vi "Facade.vi"(0 "Data In":T5={"Format"=0, "Stimulus"={"Destination"="", "Rep rate (/sec)"=0.0, "Alternate Polarity"=FALSE, "Duration (ms)"=0.0, "Ramp (ms)"=16.0, "Fs (Hz)"=5.0, "Frame size (s)"=0.0}, "Sequence"={"Freq"={"Expression"="", "Step"=80}, "Level"={"Start (dB)"=20, "Stop (dB)"=80, "Step (dB)"=5}, "Order"=enum."Interleaved"}, "Response"={"Gain"=10000.0, "Averages"=512, "Window (ms)"=8.5, "Fs (Hz)"=25000.0, "Save raw"=FALSE}, "Reject"=0.0} {"Sequence"."Level"."Start (dB)" step=5; "Response"."Window (ms)" format="%.2f"}, 2 "Display State In":T3, 3 "Container State":T4) -> (6 "Data Out":T5={"Format"=0, "Stimulus"={"Destination"="", "Rep rate (/sec)"=0.0, "Alternate Polarity"=FALSE, "Duration (ms)"=0.0, "Ramp (ms)"=16.0, "Fs (Hz)"=5.0, "Frame size (s)"=0.0}, "Sequence"={"Freq"={"Expression"="", "Step"=80}, "Level"={"Start (dB)"=20, "Stop (dB)"=80, "Step (dB)"=5}, "Order"=enum."Interleaved"}, "Response"={"Gain"=10000.0, "Averages"=512, "Window (ms)"=8.5, "Fs (Hz)"=25000.0, "Save raw"=FALSE}, "Reject"=0.0} {"Sequence"."Level"."Start (dB)" step=5; "Response"."Window (ms)" format="%.2f"}, 7 "Display State Out":T3, 8 "Action":T2)   [LabVIEW 2020, in "FABR-Parameters.xctl"]
uses:
  FABR-Parameters.xctl
  Data.vi
  FABR-Stimulus.ctl
  FABR-Sequence.ctl
  FABR-Order.ctl
  FABR-Response.ctl
  <vilib>/_xctls/Container State.ctl
  State.vi
  <vilib>/_xctls/Action.ctl
  epl-vi-lib/Utility VIs/Buttons/KCheckmarkBoolean 2.ctl
  8ab337da-13bf-40eb-afaf-d46579a93e22.vi
  <vilib>/Comparison/Equal/Equal Functor/Equal Functor.lvclass
  <vilib>/_xctls/XControlSupport.lvlib
panel:
  in  "Order":enum16{"Interleaved"}(ring)
  in  "Window (ms)":sgl=8.5 format="%.2f"
  in  "Averages":i32=512
  in  "Gain":i32=10000
  in  "Step":i32
  in  "Expr":string caption="Frequency"
  in  "Alternate Polarity":T1
  in  "Rep rate (/sec)":dbl=30.0
  in  "Step (dB)":i32=5
  in  "Max (dB)":i32=80
  in  "Min (dB)":i32=20 caption="Level" step=5
  in  "Destination":u16(ring)=1 items=["Right ear", "Left ear"]
  # "Stimulus"
  # "Response"
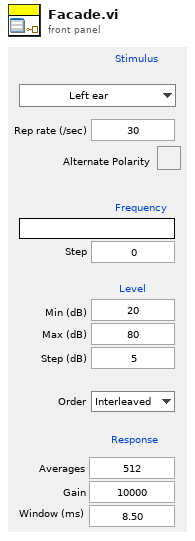
[diagram p1: front panel]
types:
  T1 = typedef "KCheckmarkBoolean 2.ctl" = bool
  T2 = typedef "XControlSupport.lvlib/Action.ctl" = cluster{"Data Changed?":bool, "State Changed?":bool, "Action Name":string}
  T3 = typedef "FABR-Parameters.xctl/State.vi" = cluster{"action":string, "destinations":string[]}
  T4 = typedef "XControlSupport.lvlib/Container State.ctl" = cluster{"Indicator?":bool, "Run Mode?":bool, " Refnum":refnum<vi>}
  T5 = typedef "FABR-Parameters.xctl/Data.vi" = cluster{"Format":i32, "Stimulus":T6, "Sequence":T7, "Response":T9, "Reject":dbl}
  T6 = typedef "FABR-Stimulus.ctl" = cluster{"Destination":string, "Rep rate (/sec)":dbl, "Alternate Polarity":bool, "Duration (ms)":dbl, "Ramp (ms)":dbl, "Fs (Hz)":dbl, "Frame size (s)":dbl}
  T7 = typedef "FABR-Sequence.ctl" = cluster{"Freq":cluster{"Expression":string, "Step":i32}, "Level":cluster{"Start (dB)":i32, "Stop (dB)":i32, "Step (dB)":i32}, "Order":T8}
  T8 = typedef "FABR-Order.ctl" = enum16{"Interleaved"}
  T9 = typedef "FABR-Response.ctl" = cluster{"Gain":dbl, "Averages":i32, "Window (ms)":sgl, "Fs (Hz)":dbl, "Save raw":bool}
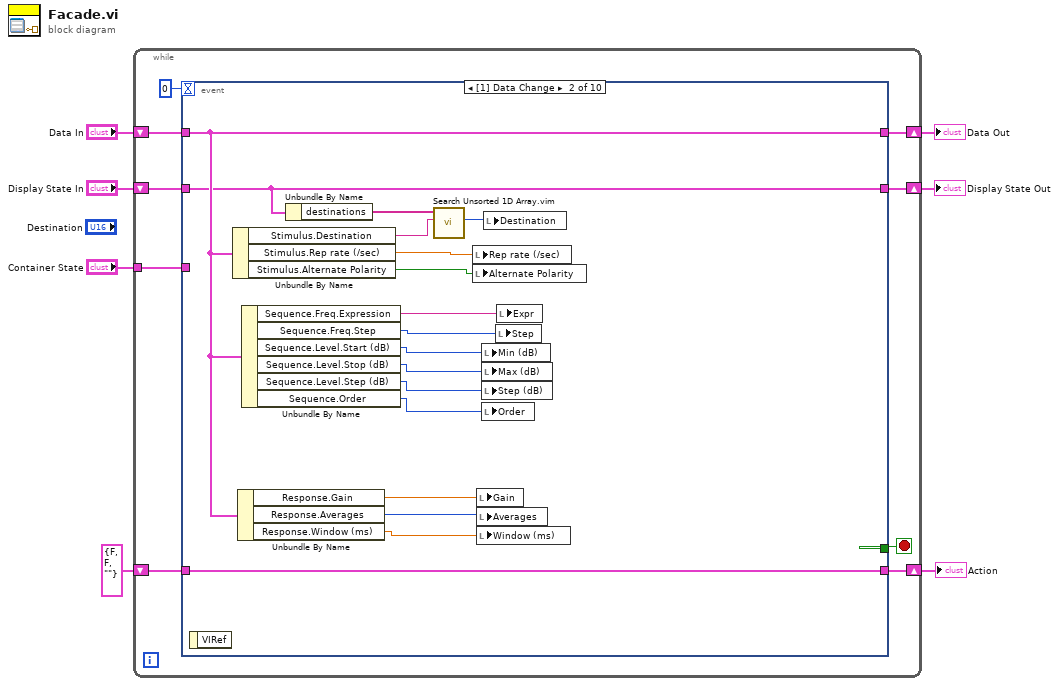
[diagram p0: block diagram]
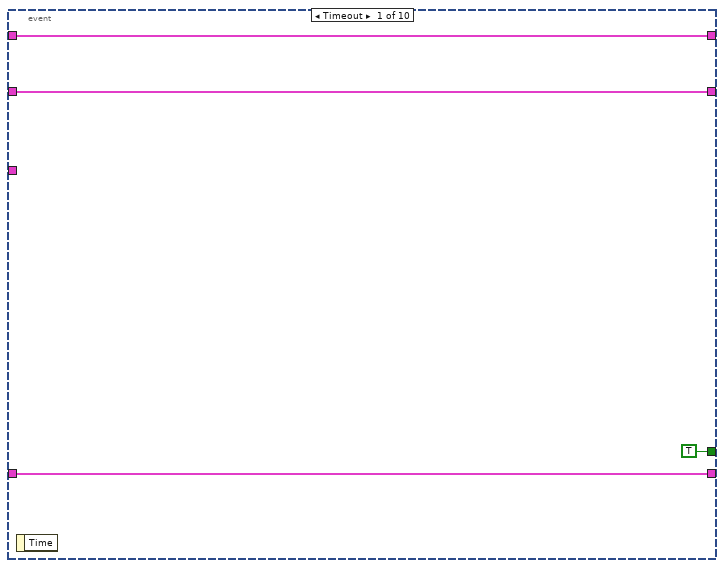
[diagram p2: hidden frame]
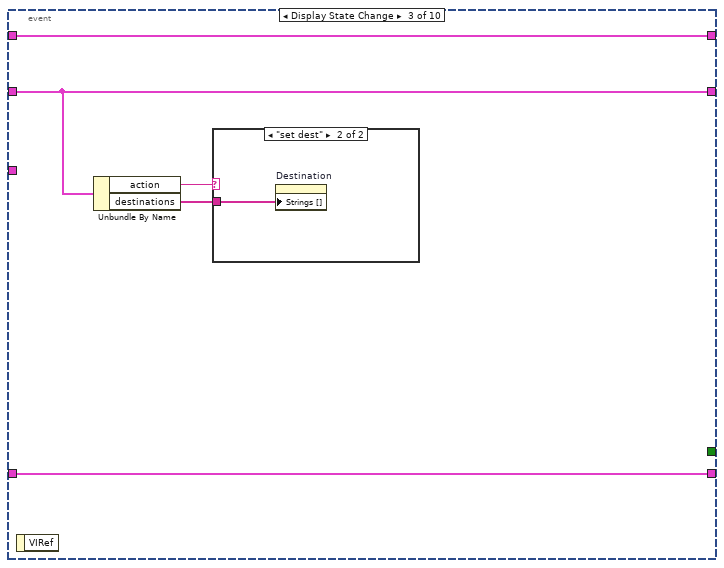
[diagram p3: hidden frame]
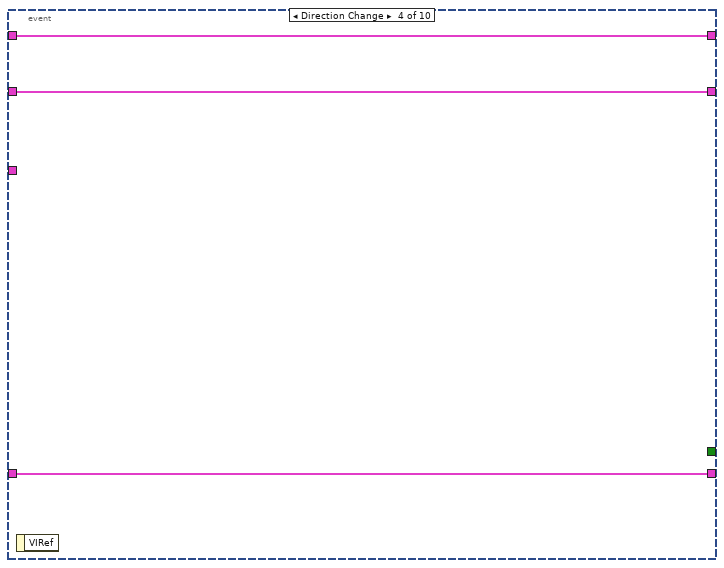
[diagram p5: hidden frame]
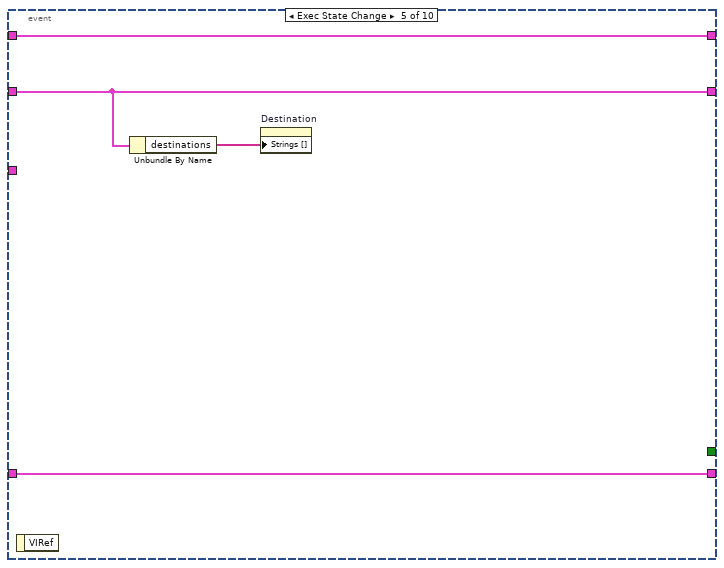
[diagram p6: hidden frame]
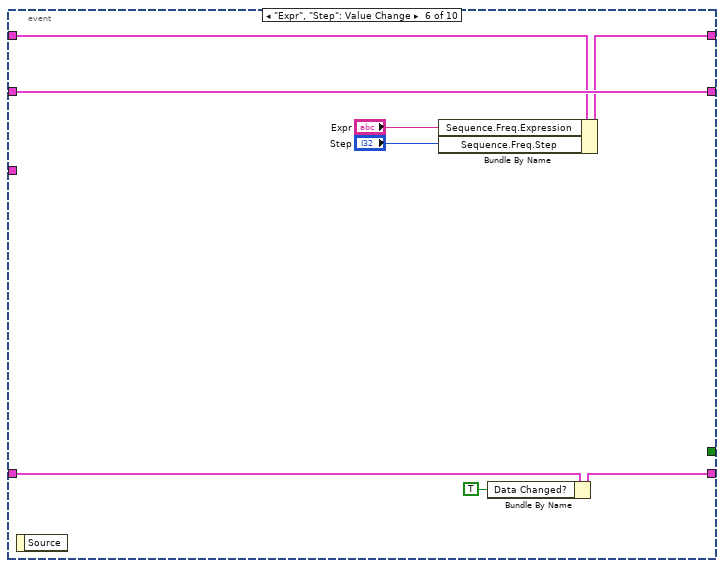
[diagram p7: hidden frame]
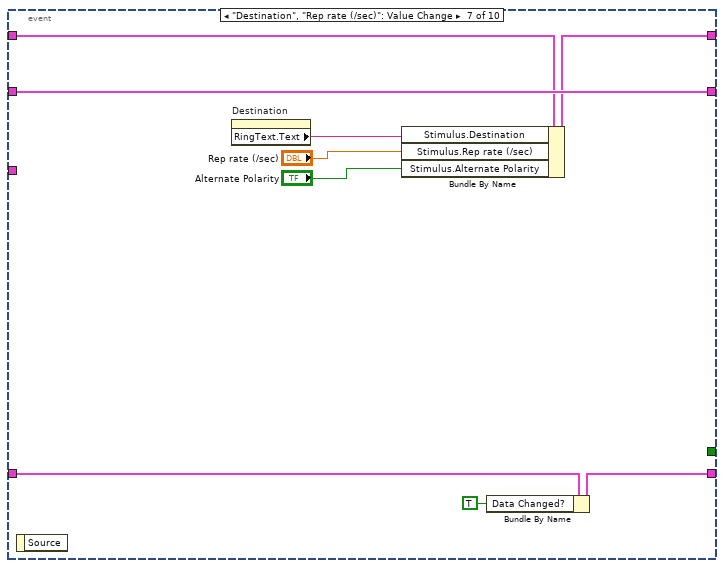
[diagram p8: hidden frame]
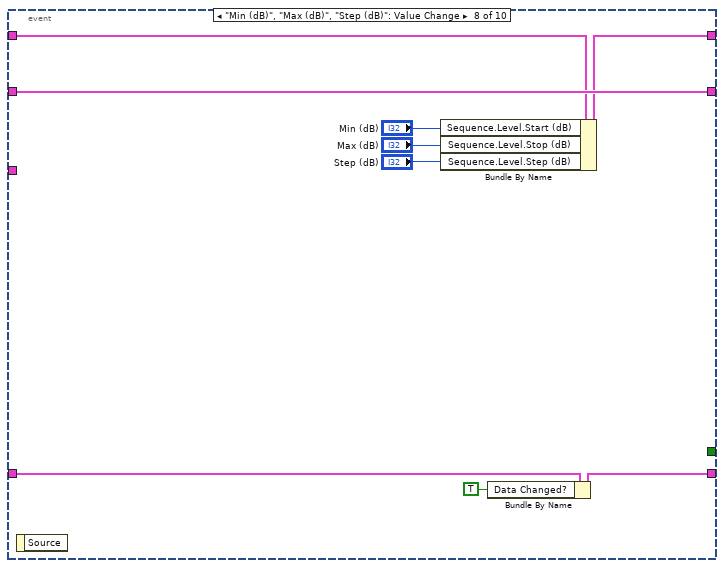
[diagram p9: hidden frame]
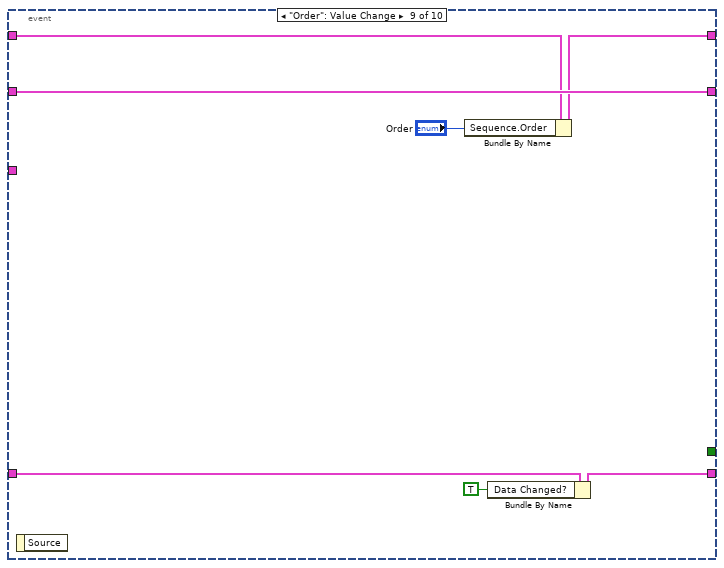
[diagram p10: hidden frame]
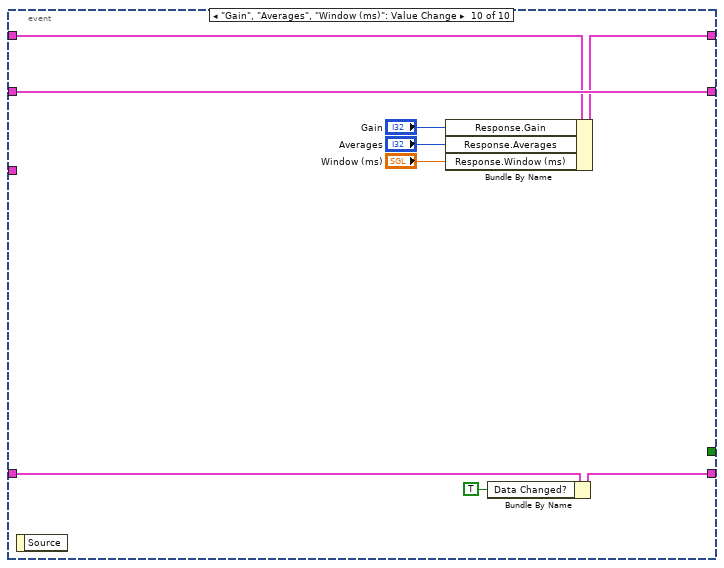
[diagram p11: hidden frame]
diagram:
  n1 = while {
    shift-right: [w15] -> w4
    shift-left: "Display State In" -> [w16]
    tunnel: "Container State" -> [w12]
    shift-right: [w10] -> w7
    shift-left: "Data In" -> [w11]
    shift-right: [w8] -> w2
    shift-left: T2 {"Data Changed?"=FALSE, "State Changed?"=FALSE, "Action Name"=""} ("Action") -> [w9]
    stop <- w14 stop-if-true
    n2 = event shown="[1] Data Change" {
      selector: _ -> [_ _ _ _ _ _ _ _ _ _]
      dyn-events: _ -> [_ _ _ _ _ _ _ _ _ _]
      timeout: 0 -> [_ _ _ _ _ _ _ _ _ _]
      tunnel: w16 -> [w18 w24 w40 w46 w48 w58 w67 w76 w83 w92]
      tunnel: [w18 w24 w40 w46 w48 w58 w67 w76 w83 w92] -> w15
      tunnel: [TRUE _ _ _ _ _ _ _ _ _] -> w14
      tunnel: w12 -> [_ _ _ _ _ _ _ _ _ _]
      tunnel: w11 -> [w17 w28 w42 w45 w50 w57 w66 w75 w82 w91]
      tunnel: [w17 w28 w42 w45 w50 w53 w62 w71 w78 w87] -> w10
      tunnel: [w19 w37 w41 w44 w49 w55 w64 w73 w80 w89] -> w8
      tunnel: w9 -> [w19 w37 w41 w44 w49 w56 w65 w74 w81 w90]
      event Timeout {
        n3 = event-data() -> ()  [unwired: 1 in, 1 out]
      }
      event Data Change {
        n4 = event-data() -> ()  [unwired: 1 in, 1 out]
        n5 = Unbundle By Name(w28) -> ("Stimulus.Destination"=w22:string, "Stimulus.Rep rate (/sec)"=w36:dbl, "Stimulus.Alternate Polarity"=w35:bool)
        n6 = Unbundle By Name(w28) -> ("Response.Gain"=w27:dbl, "Response.Averages"=w26:i32, "Response.Window (ms)"=w25:sgl)
        n7 = Unbundle By Name(w28) -> ("Sequence.Freq.Expression"=w34:string, "Sequence.Freq.Step"=w33:i32, "Sequence.Level.Start (dB)"=w32:i32, "Sequence.Level.Stop (dB)"=w31:i32, "Sequence.Level.Step (dB)"=w30:i32, "Sequence.Order"=w29:T8)
        n8 = Unbundle By Name(w24) -> ("destinations"=w23:string[])
        n9 = call "Search Unsorted 1D Array.vim"("element"=w22, "unsorted 1D array"=w23) -> ("index of element"=w21:i32)  [unwired: 9 in]
        n10 = local write "Rep rate (/sec)"(w36) -> ()
        n11 = local write "Alternate Polarity"(w35) -> ()
        n12 = local write "Gain"(w27) -> ()
        n13 = local write "Averages"(w26) -> ()
        n14 = local write "Window (ms)"(w25) -> ()
        n15 = local write "Min (dB)"(w32) -> ()
        n16 = local write "Max (dB)"(w31) -> ()
        n17 = local write "Step (dB)"(w30) -> ()
        n18 = local write "Order"(w29) -> ()
        n19 = local write "Destination"(w21) -> ()
        n20 = local write "Step"(w33) -> ()
        n21 = local write "Expr"(w34) -> ()
      }
      event Display State Change {
        n22 = event-data() -> ()  [unwired: 1 in, 1 out]
        n23 = Unbundle By Name(w40) -> ("action"=w39:string, "destinations"=w38:string[])
        n24 = case shown="\"set dest\"" w39 {
          tunnel: w38 -> [_ w43]
          frame Default {
          }
          frame "set dest" {
            n25 = property on="Destination" class="Ring (strict)"("Strings []"=w43) -> ()  [unwired: 2 in, 2 out]
          }
        }
      }
      event Direction Change {
        n26 = event-data() -> ()  [unwired: 1 in, 1 out]
      }
      event Exec State Change {
        n27 = event-data() -> ()  [unwired: 1 in, 1 out]
        n28 = Unbundle By Name(w48) -> ("destinations"=w47:string[])
        n29 = property on="Destination" class="Ring (strict)"("Strings []"=w47) -> ()  [unwired: 2 in, 2 out]
      }
      event "Expr", "Step": Value Change {
        n30 = event-data() -> ()  [unwired: 1 in, 1 out]
        n31 = Bundle By Name(cluster=w57, "Sequence.Freq.Expression"="Expr", "Sequence.Freq.Step"="Step") -> (w53:T5)
        n32 = Bundle By Name(cluster=w56, "Data Changed?"=TRUE) -> (w55:T2)
      }
      event "Destination", "Rep rate (/sec)": Value Change {
        n33 = event-data() -> ()  [unwired: 1 in, 1 out]
        n34 = property on="Destination" class="Ring (strict)"() -> ("RingText.Text"=w61:string)  [unwired: 2 in, 2 out]
        n35 = Bundle By Name(cluster=w66, "Stimulus.Destination"=w61, "Stimulus.Rep rate (/sec)"="Rep rate (/sec)", "Stimulus.Alternate Polarity"="Alternate Polarity") -> (w62:T5)
        n36 = Bundle By Name(cluster=w65, "Data Changed?"=TRUE) -> (w64:T2)
      }
      event "Min (dB)", "Max (dB)", "Step (dB)": Value Change {
        n37 = event-data() -> ()  [unwired: 1 in, 1 out]
        n38 = Bundle By Name(cluster=w75, "Sequence.Level.Start (dB)"="Min (dB)", "Sequence.Level.Stop (dB)"="Max (dB)", "Sequence.Level.Step (dB)"="Step (dB)") -> (w71:T5)
        n39 = Bundle By Name(cluster=w74, "Data Changed?"=TRUE) -> (w73:T2)
      }
      event "Order": Value Change {
        n40 = event-data() -> ()  [unwired: 1 in, 1 out]
        n41 = Bundle By Name(cluster=w82, "Sequence.Order"="Order") -> (w78:T5)
        n42 = Bundle By Name(cluster=w81, "Data Changed?"=TRUE) -> (w80:T2)
      }
      event "Gain", "Averages", "Window (ms)": Value Change {
        n43 = event-data() -> ()  [unwired: 1 in, 1 out]
        n44 = Bundle By Name(cluster=w91, "Response.Gain"="Gain", "Response.Averages"="Averages", "Response.Window (ms)"="Window (ms)") -> (w87:T5)
        n45 = Bundle By Name(cluster=w90, "Data Changed?"=TRUE) -> (w89:T2)
      }
    }
  }
  "Display State Out" <- w4
  "Data Out" <- w7
  "Action" <- w2
